vi "Miniquads.contents.vi"   [LabVIEW 2014, in "Miniquads.lvlib"]
doc: "Contains \"all\" VIs. Required for building applications."
uses:
  Miniquads.lvlib
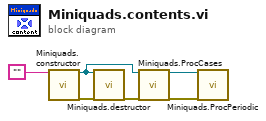
[diagram p0: block diagram]
diagram:
  n1 = call "Miniquads.constructor.vi"("name"="") -> ("i ref out"=w5:refnum<vi>, "error out"=w3:errorcluster)  [unwired: 16 in, 1 out]
  n2 = call "Miniquads.destructor.vi"("i ref in"=w5, "error in (no error)"=w3) -> ("error out"=w2:errorcluster)  [unwired: 17 in]
  n3 = call "Miniquads.ProcCases.vi"("i ref in"=w5, "error in (no error)"=w2) -> ("i ref out"=w4:refnum<vi>, "error out"=w1:errorcluster)  [unwired: 15 in, 1 out]
  n4 = call "Miniquads.ProcPeriodic.vi"("i ref in"=w4, "error in (no error)"=w1) -> ()  [unwired: 15 in, 3 out]
